vi "Update Listbox.vi"(6 "Clear":bool, 10 "Route Target":string, 11 "referencein":refnum<vi>) -> (3 "reference out":refnum<vi>)   [LabVIEW 2019, in "MLTFNC.lvlib" / "MLTFNC.lvclass"]
uses:
  Library/MLTFNC.lvclass
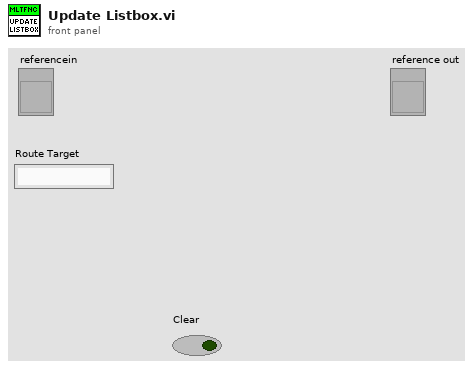
[diagram p1: front panel]
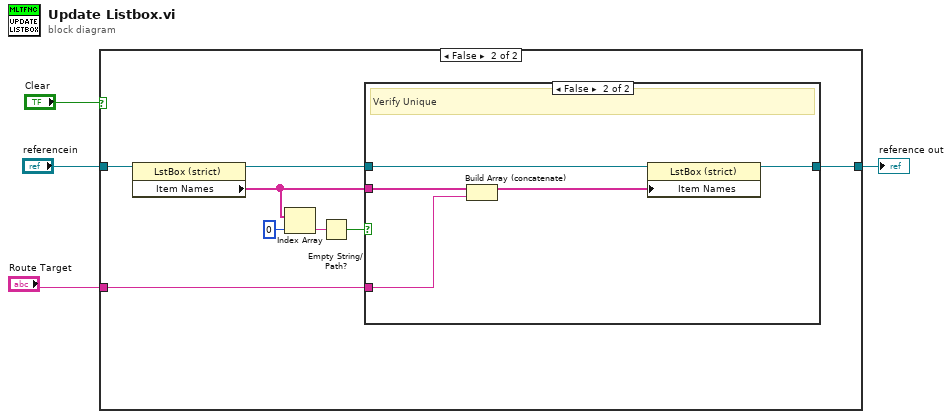
[diagram p0: block diagram]
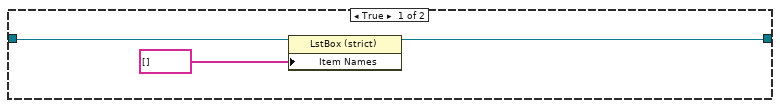
[diagram p2: hidden frame]
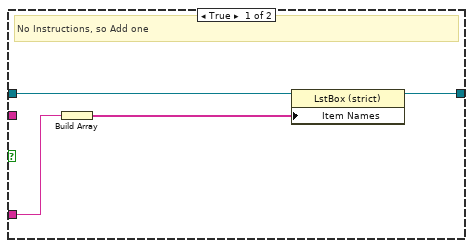
[diagram p3: hidden frame]
diagram:
  n1 = case shown="False" "Clear" {
    tunnel: [w6 w14] -> w4
    tunnel: "Route Target" -> [_ w13]
    tunnel: "referencein" -> [w7 w12]
    frame True {
      n2 = property class="LstBox (strict)"(reference=w7, "Item Names"=string[] []) -> (reference out=w6:refnum<vi>)  [unwired: 1 in, 1 out]
    }
    frame False {
      n3 = property class="LstBox (strict)"(reference=w12) -> (reference out=w15:refnum<vi>, "Item Names"=w11:string[])  [unwired: 1 in, 1 out]
      n4 = Index Array(array=w11, index=0 ("index (row)")) -> (element=w9:string)
      n5 = Empty String/Path?(string/path=w9) -> (empty?=w8:bool)
      n6 = case shown="False" w8 {
        tunnel: w15 -> [w19 w24]
        tunnel: [w18 w23] -> w14
        tunnel: w13 -> [w17 w22]
        tunnel: w11 -> [_ w20]
        frame True {
          # "No Instructions, so Add one"
          n7 = Build Array(w17) -> (w16:string[])
          n8 = property class="LstBox (strict)"(reference=w19, "Item Names"=w16) -> (reference out=w18:refnum<vi>)  [unwired: 1 in, 1 out]
        }
        frame False {
          # "Verify Unique"
          n9 = Build Array (concatenate)(w20, w22) -> (w21:string[])
          n10 = property class="LstBox (strict)"(reference=w24, "Item Names"=w21) -> (reference out=w23:refnum<vi>)  [unwired: 1 in, 1 out]
        }
      }
    }
  }
  "reference out" <- w4
